vi "runnerFrontEnd.vi"(6 "ExperimentControlEvents":refnum<class "ExperimentControlEvents.lvclass">, 8 "error in (no error)":errorcluster, 9 "deviceDataBase":refnum<class "deviceDataBase.lvclass">, 10 "HWControllerEvents":refnum<class "HWControllerEvents.lvclass">, 11 "Views.lvlib:ExperimentControl.lvlib:ExperimentRunner in":refnum<class "ExperimentRunner.lvclass">) -> (0 "error out":errorcluster, 3 "Views.lvlib:ExperimentControl.lvlib:ExperimentRunner out":refnum<class "ExperimentRunner.lvclass">)   [LabVIEW 2009, in "Views.lvlib" / "ExperimentControl.lvlib" / "ExperimentRunner.lvclass"]
doc: "Experiment Runner Front End.\n\nThis is the user interface to control the expeirment. I.e. Run scripts and control the hardware state."
uses:
  ExperimentRunner.lvclass
  Hal/HWController/HWControllerEvents/HWControllerEvents.lvclass
  Tools/DatabaseHelpers/DbConnection/DeviceDataBase/deviceDataBase.lvclass
  Events/ExperimentControlEvents.lvclass
  ExperimentRunner.lvclass/ExperimentRunner.ctl
  Tools/SettingsProcessors/Compiler/Compiler.lvclass
  ScriptEditor/ScriptEditorV2/ScriptEditorV2.lvclass
  EventEditor/StaticOutputEditor/StaticOutputEditor.lvclass
  ScriptEditor/ScriptEdEvents/ScriptEdEvents.lvclass
  Tools/Filing/FileNeologist/FileNeologist.lvclass
  <vilib>/Utility/error.llb/DialogType.ctl
  Tools/DatabaseHelpers.lvlib
  Tools/Filing.lvlib
panel:
  in  "experimentFunction":enum16{"runListOnce", "loopOverList"}(ring)
  out "runningScriptName":string
  in  "HW Loop?":bool
  in  "refreshDatabase":bool
  in  "staticOutput":bool
  in  "stop":bool
  in  "runScript":bool
  in  "viewScript":bool
  in  "removePath":bool
  in  "addPath":bool
  out "status":T1(ring)
  in  "Listbox":i32(listbox)
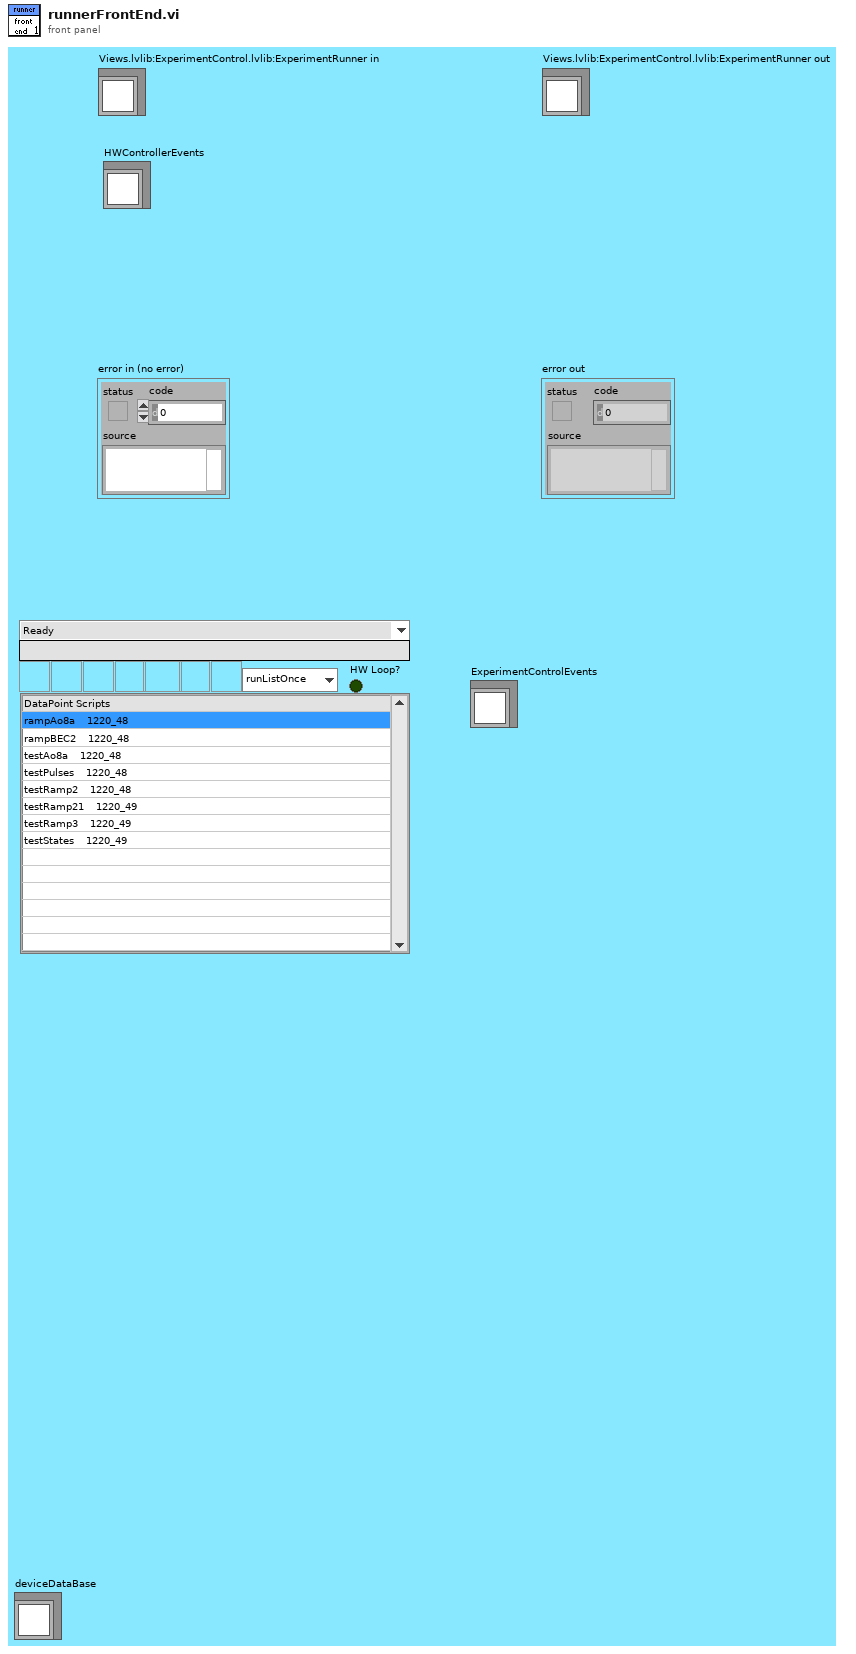
[diagram p1: front panel]
types:
  T1 = enum16{"Ready", "Compiling", "Configured", "Running", "Stopping", "Unresolved Error"}
  T2 = enum16{"start", "stop", "statusInquiry", "configure", "resetError", "resourcesInquiry", "reserveResources", "initialise", "resetAllChannels", "staticUpdate", "close", "HWStatus", "error", "resourcesAvailable", "resourcesReserved", "compilerError", "compiledScript", "compilingScript", "runScript", "configureCompiledScript"}
  T3 = enum16{"start", "stop", "statusInquiry", "configure", "resetError", "resourcesInquiry", "reserveResources", "initialise", "resetAllChannels", "staticUpdate", "close", "HWStatus", "error", "resourcesAvailable", "resourcesReserved"}
  T4 = enum16{"start", "stop", "statusInquiry", "configure", "resetError", "resourcesInquiry", "reserveResources", "initialise", "resetAllChannels", "staticUpdate", "close", "HWStatus", "error", "resourcesAvailable", "resourcesReserved", "compilerError", "compiledScript", "compilingScript", "runScript", "configureCompiledScript", "restartCompiler"}
  T5 = cluster{"incomingEventTypes":cluster{"start":cluster{"Boolean":bool}, "stop":cluster{"Boolean":bool}, "statusInquiry":cluster{"Boolean":bool}, "configure":cluster{"DPScriptPath":path, "TimeStamp":string, "HWLoop?":bool}, "resetError":cluster{"Boolean":bool}, "resourcesInquiry":cluster{"Boolean":bool}, "reserveResources":cluster{"HWList":string[]}, "initialise":cluster{"HWList":string[]}, "close":cluster{"Boolean":bool}, "resetAllChannels":cluster{"Boolean":bool}, "staticChannelUpdate":cluster{"channel_address":string, "calibratedValue":dbl}, "runScript":cluster{"DPScriptPath":path, "TimeStamp":string, "HWLoop?":bool}, "compilingScript":cluster{"Path":path}, "compiledScript":cluster{"Path":path, "timeCompileAt":string}, "compilerError":cluster{"Path":path}, "configureCompiledScript":cluster{"DPScriptPath":path, "TimeStamp":string, "HWLoop?":bool, "CompiledScript":cluster{"ScriptListCompiler.lvclass":refnum<class "ScriptListCompiler.lvclass">, "aoChannels":refnum<class "AnalogOutput.lvclass">[], "doChannels":refnum<class "DigitalOutput.lvclass">[], "rfChannels":refnum<class "DDSOutput.lvclass">[]}}, "restartCompiler":cluster{"restart":bool}, "staticRfChannelUpdate":cluster{"channel_address":string, "Output":cluster{"Frequency(MHz)":dbl, "Amplitude":dbl, "Phase":dbl, "OutputForm":enum16{"Sine", "Square", "Triangle", "Arbitrary"}}}}, "outgoingEventTypes":cluster{"HWStatus":cluster{"status":enum16{"Ready", "Compiling", "Configured", "Running", "Stopping", "Unresolved Error"}}, "error":cluster{"error out":errorcluster}, "resourcesAvailable":cluster{"availableHWList":string[], "reservedHWList":string[]}, "resourcesReserved":cluster{"reservedHWList":string[]}}}
  T6 = cluster{"open":cluster{"Path":path}, "close":cluster{"Boolean":bool}, "save":cluster{"Path":path}}
  T7 = cluster{"eventId":enum16{"Open", "Save", "Close"}, "close":cluster{"Boolean":bool}}
  T8 = cluster{"eventId":enum16{"start", "stop", "statusInquiry", "configure", "resetError", "resourcesInquiry", "reserveResources", "initialise", "resetAllChannels", "staticUpdate", "close", "HWStatus", "error", "resourcesAvailable", "resourcesReserved", "compilerError", "compiledScript", "compilingScript", "runScript", "configureCompiledScript"}, cluster{bool}}
  T9 = cluster{"eventId":enum16{"Open", "Save", "Close"}, "open":cluster{"Path":path}}
  T10 = typedef "eventsource.ctl" = u32
  T11 = enum16{"start", "stop", "statusInquiry", "configure", "resetError", "resourcesInquiry", "reserveResources", "initialise", "resetAllChannels", "staticUpdate", "close", "HWStatus", "error", "resourcesAvailable", "resourcesReserved", "compilerError", "compiledScript", "compilingScript", "runScript", "configureCompiledScript", "restartCompiler", "staticRfChannelUpdate"}
  T12 = cluster{"status":enum16{"Ready", "Compiling", "Configured", "Running", "Stopping", "Unresolved Error"}}
  T13 = typedef "DialogType.ctl" = u16
  T14 = cluster{"eventId":enum16{"start", "stop", "statusInquiry", "configure", "resetError", "resourcesInquiry", "reserveResources", "initialise", "resetAllChannels", "staticUpdate", "close", "HWStatus", "error", "resourcesAvailable", "resourcesReserved"}, "resetError":cluster{"Boolean":bool}}
  T15 = cluster{"eventId":enum16{"start", "stop", "statusInquiry", "configure", "resetError", "resourcesInquiry", "reserveResources", "initialise", "resetAllChannels", "staticUpdate", "close", "HWStatus", "error", "resourcesAvailable", "resourcesReserved"}, cluster{bool}}
  T16 = typedef "LVPoint32TypeDef.ctl" = cluster{"Horizontal":i32, "Vertical":i32}
  T17 = cluster{"eventId":enum16{"start", "stop", "statusInquiry", "configure", "resetError", "resourcesInquiry", "reserveResources", "initialise", "resetAllChannels", "staticUpdate", "close", "HWStatus", "error", "resourcesAvailable", "resourcesReserved", "compilerError", "compiledScript", "compilingScript", "runScript", "configureCompiledScript", "restartCompiler"}, cluster{bool}}
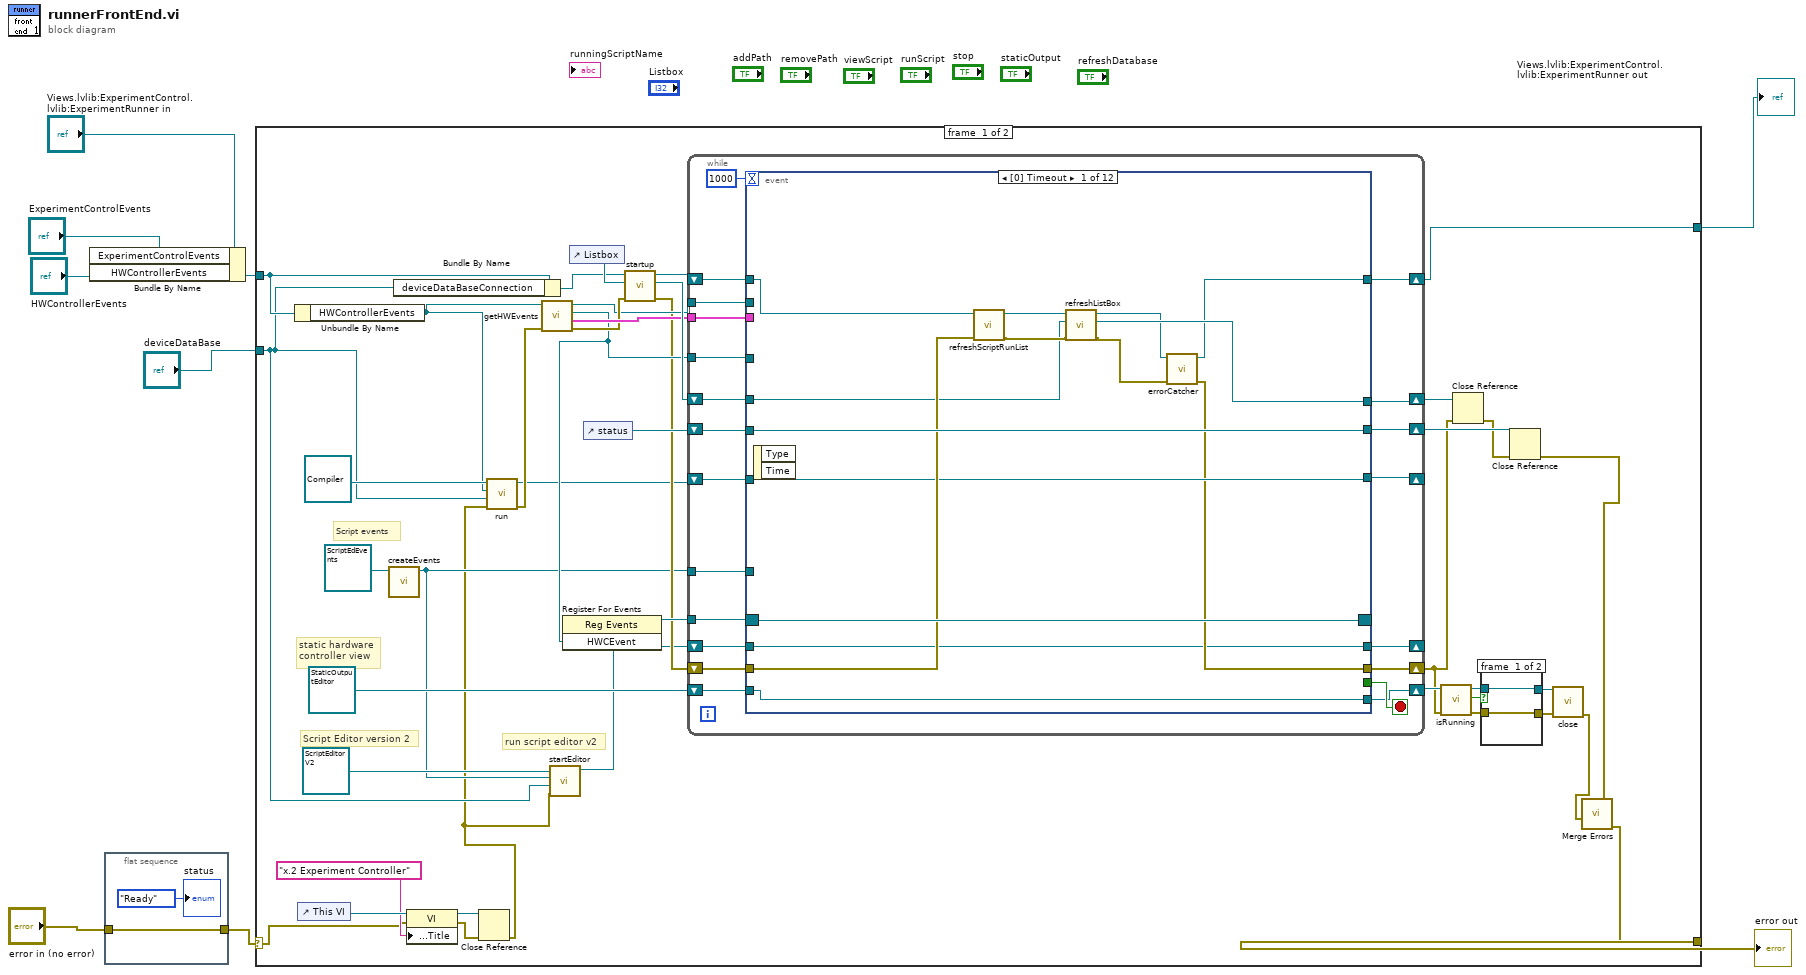
[diagram p0: block diagram]
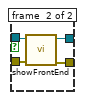
[diagram p2: hidden frame]
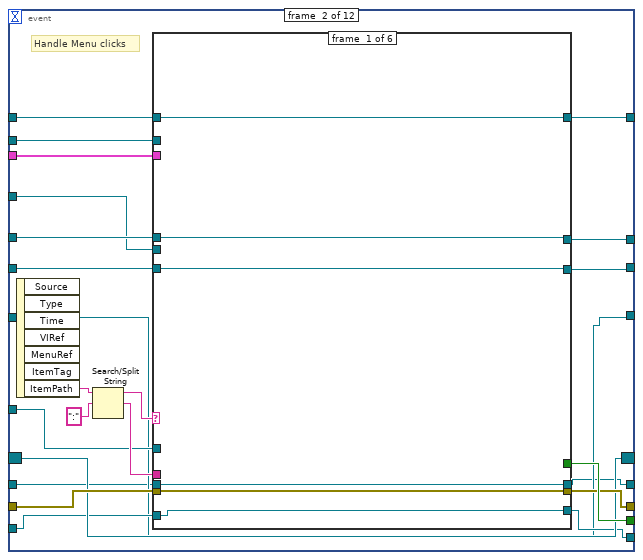
[diagram p3: hidden frame]
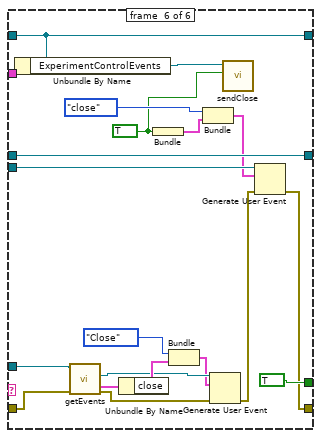
[diagram p9: hidden frame]
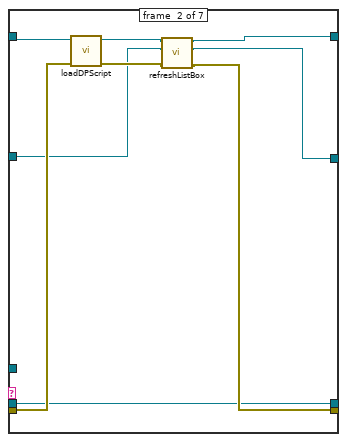
[diagram p17: hidden frame]
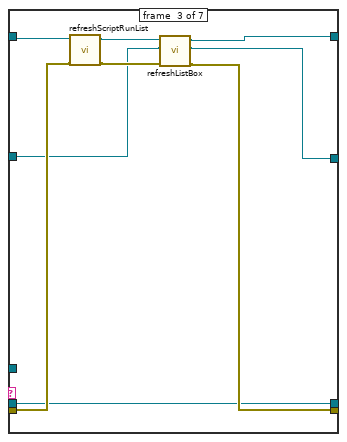
[diagram p18: hidden frame]
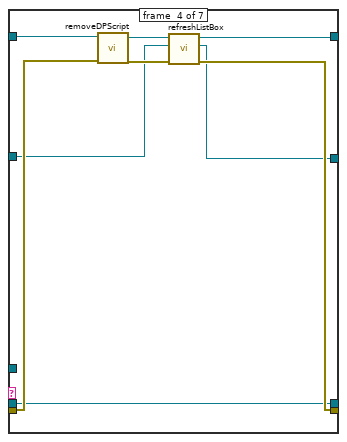
[diagram p19: hidden frame]
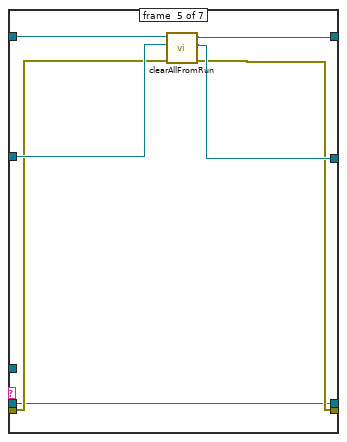
[diagram p20: hidden frame]
diagram:
  n1 = Bundle By Name(cluster="Views.lvlib:ExperimentControl.lvlib:ExperimentRunner in", "ExperimentControlEvents"="ExperimentControlEvents", "HWControllerEvents"="HWControllerEvents") -> (w5:refnum<class "ExperimentRunner.lvclass">)
  n2 = flat-sequence {
    tunnel: "error in (no error)" -> [w10]
    tunnel: [w10] -> w2
    frame #0 {
      "status" <- T1."Ready" ("status")
    }
  }
  n3 = case shown="No Error" w2 {
    selector: w2 -> [w28 w688]
    tunnel: [w41 w688] -> w9
    tunnel: [w32 w687] -> w8
    tunnel: w5 -> [w36 w687]
    tunnel: "deviceDataBase" -> [w14 _]
    frame #0 {
      # "run script editor v2"
      # "Script Editor version 2"
      # "Script events"
      # "static hardware\ncontroller view"
      n4 = Unbundle By Name(w36) -> ("HWControllerEvents"=w29:refnum<class "HWControllerEvents.lvclass">)
      n5 = control-ref of="This VI"() -> (w40:refnum<vi>)
      n6 = call-dynamic "createEvents.vi"("ScriptEdEvents in"=refnum<class "ScriptEdEvents.lvclass"> refnum ("Views.lvlib:SciptEditor.lvlib:ScriptEdEvents.lvclass")) -> ("ScriptEdEvents out"=w15:refnum<class "ScriptEdEvents.lvclass">)  [unwired: 9 in, 1 out]
      n7 = Bundle By Name(cluster=w36, "deviceDataBaseConnection"=w14) -> (w35:refnum<class "ExperimentRunner.lvclass">)
      n8 = property class="VI"(reference=w40, error in=w28, "Front Panel.Title"="x.2 Experiment Controller") -> (reference out=w38:refnum<vi>, error out=w37:errorcluster)
      n9 = Close Reference(reference=w38, error in (no error)=w37) -> (error out=w13:errorcluster)
      n10 = call "run.vi"("error in (no error)"=w13, "deviceDataBase"=w14, "HWControllerEvents"=w29, "Compiler in"=refnum<class "Compiler.lvclass"> refnum) -> ("error out"=w27:errorcluster, "Compiler out"=w26:refnum<class "Compiler.lvclass">)  [unwired: 6 in]
      n11 = call-dynamic "getHWEvents.vi"("error in (no error)"=w27, "HWControllerEvents in"=w29) -> ("error out"=w47:errorcluster, "eventDataTypes"=w48:T5, "HWCEvent"=w46:refnum<user-event>, "HWControllerEvents out"=w34:refnum<class "HWControllerEvents.lvclass">)  [unwired: 6 in]
      n12 = call "startEditor.vi"("error in (no error)"=w13, "deviceDataBase"=w14, "ScriptEdEvents"=w15, "ScriptEditorV2 in"=refnum<class "ScriptEditorV2.lvclass"> refnum ("Views.lvlib:SciptEditor.lvlib:ScriptEditorV2.lvclass")) -> ("ScriptEditorV2 out"=w12:refnum<class "ScriptEditorV2.lvclass">)  [unwired: 6 in, 1 out]
      n13 = register-events(w46) -> (reference out=w49:refnum<event-registration>)  [unwired: 2 in, 1 out]
      n14 = control-ref of="Listbox"() -> (w51:refnum<vi>)
      n15 = control-ref of="status"() -> (w45:refnum<vi>)
      n16 = call "startup.vi"("error in (no error)"=w47, "Listbox in"=w51, "ExperimentRunner in"=w35) -> ("error out"=w31:errorcluster, "Listbox out"=w50:refnum<vi>, "ExperimentRunner out"=w52:refnum<class "ExperimentRunner.lvclass">)  [unwired: 6 in]
      n17 = while {
        shift-right: [w79] -> w32
        shift-left: w52 -> [w66]
        shift-right: [w78] -> w24
        shift-left: w31 -> [w65]
        shift-right: [w77] -> w53
        shift-left: w50 -> [w67]
        tunnel: w49 -> [w76]
        tunnel: w48 -> [w75]
        tunnel: w46 -> [w74]
        shift-right: [w72] -> w44
        shift-left: w45 -> [w73]
        tunnel: w15 -> [w71]
        tunnel: w34 -> [w70]
        shift-right: [w68] -> w25
        shift-left: refnum<class "StaticOutputEditor.lvclass"> refnum ("Views.lvlib:SciptEditor.lvlib:StaticOutputEditor.lvclass") -> [w69]
        shift-right: [w62] -> _
        shift-left: w26 -> [w63]
        shift-right: [w61] -> _
        shift-left: w12 -> [w60]
        stop <- w80 stop-if-true
        n18 = event shown="[0] Timeout" {
          selector: w76 -> [w94 w107 w389 _ _ w564 w577 w584 w618 w631 w639 w675]
          dyn-events: [w94 w107 w389 _ _ w564 w577 w584 w618 w631 w639 w675] -> _
          timeout: 1000 -> [_ _ _ _ _ _ _ _ _ _ _ _]
          tunnel: [_ w118 _ TRUE _ _ _ _ _ _ _ _] -> w80
          tunnel: w66 -> [w92 w113 w383 w518 w547 w568 w581 w596 w614 w625 w646 w685]
          tunnel: [w82 w112 w382 w517 w546 w562 w575 w596 w613 w624 w646 w684] -> w79
          tunnel: [w84 w110 w390 w522 w554 w558 w571 w592 w611 w626 w644 w664] -> w78
          tunnel: w65 -> [w91 w111 w391 w521 w543 w565 w579 w594 w615 w627 w635 w673]
          tunnel: w67 -> [w88 w109 w381 w538 w548 w561 w574 w595 w620 w630 w641 w682]
          tunnel: [w87 w108 w380 w538 w548 w560 w573 w595 w620 w630 w641 w682] -> w77
          tunnel: w75 -> [_ w106 w392 _ _ _ _ _ _ _ _ _]
          tunnel: w74 -> [_ w105 w385 w524 _ _ _ _ _ _ _ w679]
          tunnel: w73 -> [w95 w104 w388 w537 w544 w567 w580 w585 w612 w629 w640 w681]
          tunnel: [w95 w103 w387 w537 w544 w567 w580 w585 w612 w629 w640 w681] -> w72
          tunnel: w71 -> [_ w102 _ w523 _ _ _ w593 _ _ _ _]
          tunnel: w70 -> [_ w101 _ _ _ _ _ _ _ _ w645 _]
          tunnel: w69 -> [w93 w100 w384 w536 w542 w566 w578 w591 w619 w628 w637 w683]
          tunnel: [w93 w99 w384 w536 w542 w566 w578 w591 w619 w628 w643 w683] -> w68
          tunnel: w63 -> [w86 w98 w379 w515 w541 w557 w570 w583 w610 w622 w638 w668]
          tunnel: [w86 w98 w379 w515 w541 w557 w570 w583 w610 w622 w638 w665] -> w62
          tunnel: [w81 w96 w378 w514 w540 w556 w569 w582 w609 w621 w632 w663] -> w61
          tunnel: w60 -> [w81 w97 w378 w514 w540 w556 w569 w582 w609 w621 w632 w663]
          event #0 {
            n19 = event-data() -> ()  [unwired: 1 in, 2 out]
            n20 = call "refreshScriptRunList.vi"("error in (no error)"=w91, "ExperimentRunner in"=w92) -> ("error out"=w90:errorcluster, "ExperimentRunner out"=w89:refnum<class "ExperimentRunner.lvclass">)  [unwired: 8 in]
            n21 = call "refreshListBox.vi"("error in (no error)"=w90, "Listbox"=w88, "ExperimentRunner in"=w89) -> ("error out"=w85:errorcluster, "Listbox out"=w87:refnum<vi>, "ExperimentRunner out"=w83:refnum<class "ExperimentRunner.lvclass">)  [unwired: 6 in]
            n22 = call "errorCatcher.vi"("error in (no error)"=w85, "ExperimentRunner in"=w83) -> ("error out"=w84:errorcluster, "ExperimentRunner out"=w82:refnum<class "ExperimentRunner.lvclass">)  [unwired: 8 in]
          }
          event #1 {
            # "Handle Menu clicks"
            n23 = event-data() -> ("ItemPath"=w116:string)  [unwired: 1 in, 6 out]
            n24 = Search/Split String(string=w116, search string/char (-)=":") -> (substring before match=w115:string, match + rest of string=w114:string)  [unwired: 1 in, 1 out]
            n25 = case shown="\"Scripting\"" w115 {
              tunnel: [_ w138 _ _ _ _] -> w118
              tunnel: w114 -> [_ w137 w178 w208 w299 w349]
              tunnel: w113 -> [w124 w136 w182 w212 w303 w348]
              tunnel: [w124 w135 w181 w211 w302 w347] -> w112
              tunnel: w111 -> [w123 w134 w179 w209 w300 w346]
              tunnel: [w123 w133 w180 w210 w301 w345] -> w110
              tunnel: w109 -> [w122 w132 w177 w207 w298 w344]
              tunnel: [w122 w131 w176 w206 w297 w344] -> w108
              tunnel: w106 -> [_ w130 _ _ _ _]
              tunnel: w105 -> [_ w129 _ _ _ w342]
              tunnel: w104 -> [w121 w128 w175 w205 w296 w343]
              tunnel: [w121 w128 w175 w205 w295 w343] -> w103
              tunnel: w102 -> [_ w127 _ w204 _ _]
              tunnel: w101 -> [_ _ _ _ _ w341]
              tunnel: w100 -> [w120 w126 w174 w203 w294 w340]
              tunnel: [w120 w126 w174 w203 w294 w339] -> w99
              tunnel: w97 -> [w119 w125 w173 w202 w293 w338]
              tunnel: [w119 w125 w173 w201 w293 w338] -> w96
              frame #0 {
              }
              frame #1 {
                n26 = case shown="\":Close\"" w137 {
                  tunnel: [_ _ _ _ _ TRUE] -> w138
                  tunnel: [w141 w144 w147 w150 w153 w156] -> w135
                  tunnel: w136 -> [w141 w144 w147 w150 w153 w156]
                  tunnel: w134 -> [w140 w143 w146 w149 w152 w158]
                  tunnel: [w140 w143 w146 w149 w152 w167] -> w133
                  tunnel: w132 -> [w139 w142 w145 w148 w151 w171]
                  tunnel: [w139 w142 w145 w148 w151 w171] -> w131
                  tunnel: w130 -> [_ _ _ _ _ _]
                  tunnel: w129 -> [_ _ _ _ _ w170]
                  tunnel: w127 -> [_ _ _ _ _ w166]
                  frame #0 {
                  }
                  frame #1 {
                  }
                  frame #2 {
                  }
                  frame #3 {
                  }
                  frame #4 {
                  }
                  frame #5 {
                    w154 = TRUE
                    n27 = Unbundle By Name(w156) -> ("ExperimentControlEvents"=w155:refnum<class "ExperimentControlEvents.lvclass">)
                    n28 = call-dynamic "getEvents.vi"("error in (no error)"=w158, "ScriptEdEvents in"=w166) -> ("error out"=w160:errorcluster, "eventsToScriptEd"=w165:T6, "ScriptEvent"=w162:refnum<user-event>)  [unwired: 6 in, 1 out]
                    n29 = Unbundle By Name(w165) -> ("close"=w163:cluster{"Boolean":bool})
                    n30 = Bundle(w154) -> (w169:cluster{bool})  [unwired: 1 in]
                    n31 = Bundle("eventId"=enum16{"Open", "Save", "Close"}."Close", "close"=w163) -> (w161:T7)  [unwired: 1 in]
                    n32 = Bundle("eventId"=T2."close", w169) -> (w168:T8)  [unwired: 1 in]
                    n33 = Generate User Event(user event=w162, event data cluster=w161, error in=w160) -> (error out=w159:errorcluster)  [unwired: 1 out]
                    n34 = call "sendClose.vi"("close"=w154, "ExperimentControlEvents in"=w155) -> ()  [unwired: 8 in, 2 out]
                    n35 = Generate User Event(user event=w170, event data cluster=w168, error in=w159) -> (error out=w167:errorcluster)  [unwired: 1 out]
                  }
                }
              }
              frame #2 {
                n36 = case shown="\":Paste\"" w178 {
                  tunnel: [w185 w188 w191 w194 w197 w200] -> w181
                  tunnel: w182 -> [w185 w188 w191 w194 w197 w200]
                  tunnel: [w184 w187 w190 w193 w196 w199] -> w180
                  tunnel: w179 -> [w184 w187 w190 w193 w196 w199]
                  tunnel: w177 -> [w183 w186 w189 w192 w195 w198]
                  tunnel: [w183 w186 w189 w192 w195 w198] -> w176
                  frame #0 {
                  }
                  frame #1 {
                  }
                  frame #2 {
                  }
                  frame #3 {
                  }
                  frame #4 {
                  }
                  frame #5 {
                  }
                }
              }
              frame #3 {
                n37 = case shown="\":Open Script Editor\"" w208 {
                  tunnel: [w216 w221 w229 w239 w246 w260 w276] -> w211
                  tunnel: w212 -> [w216 w225 w234 w243 w250 w260 w276]
                  tunnel: [w215 w218 w231 w240 w245 w255 w278] -> w210
                  tunnel: w209 -> [w215 w224 w233 w242 w248 w256 w282]
                  tunnel: w207 -> [w214 w220 w228 w237 w249 w261 w284]
                  tunnel: [w214 w219 w227 w236 w247 w261 w284] -> w206
                  tunnel: w204 -> [_ _ _ _ _ w257 w274]
                  tunnel: w202 -> [w213 w217 w226 w235 w244 w251 w283]
                  tunnel: [w213 w217 w226 w235 w244 w251 w280] -> w201
                  frame #0 {
                  }
                  frame #1 {
                    n38 = call "loadDPScript.vi"("error in (no error)"=w224, "ExperimentRunner in"=w225) -> ("error out"=w223:errorcluster, "ExperimentRunner out"=w222:refnum<class "ExperimentRunner.lvclass">)  [unwired: 8 in]
                    n39 = call "refreshListBox.vi"("error in (no error)"=w223, "Listbox"=w220, "ExperimentRunner in"=w222) -> ("error out"=w218:errorcluster, "Listbox out"=w219:refnum<vi>, "ExperimentRunner out"=w221:refnum<class "ExperimentRunner.lvclass">)  [unwired: 6 in]
                  }
                  frame #2 {
                    n40 = call "refreshScriptRunList.vi"("error in (no error)"=w233, "ExperimentRunner in"=w234) -> ("error out"=w232:errorcluster, "ExperimentRunner out"=w230:refnum<class "ExperimentRunner.lvclass">)  [unwired: 8 in]
                    n41 = call "refreshListBox.vi"("error in (no error)"=w232, "Listbox"=w228, "ExperimentRunner in"=w230) -> ("error out"=w231:errorcluster, "Listbox out"=w227:refnum<vi>, "ExperimentRunner out"=w229:refnum<class "ExperimentRunner.lvclass">)  [unwired: 6 in]
                  }
                  frame #3 {
                    n42 = call "removeDPScript.vi"("error in (no error)"=w242, "ExperimentRunner in"=w243) -> ("error out"=w241:errorcluster, "ExperimentRunner out"=w238:refnum<class "ExperimentRunner.lvclass">)  [unwired: 8 in]
                    n43 = call "refreshListBox.vi"("error in (no error)"=w241, "Listbox"=w237, "ExperimentRunner in"=w238) -> ("error out"=w240:errorcluster, "Listbox out"=w236:refnum<vi>, "ExperimentRunner out"=w239:refnum<class "ExperimentRunner.lvclass">)  [unwired: 6 in]
                  }
                  frame #4 {
                    n44 = call "clearAllFromRun.vi"("error in (no error)"=w248, "Listbox in"=w249, "ExperimentRunner in"=w250) -> ("error out"=w245:errorcluster, "Listbox out"=w247:refnum<vi>, "ExperimentRunner out"=w246:refnum<class "ExperimentRunner.lvclass">)  [unwired: 6 in]
                  }
                  frame #5 {
                    # "send open event to script editor"
                    n45 = Unbundle By Name(w260) -> ("scriptSelected"=w258:i32, "PathArray"=w259:path[])
                    n46 = Index Array(array=w259, index=w258) -> (element=w254:path)
                    n47 = Equal?(x=w254, y=path "") -> (x = y?=w252:bool)
                    n48 = case shown="False" w252 {
                      tunnel: w257 -> [w272 _]
                      tunnel: w256 -> [w271 w273]
                      tunnel: [w263 w273] -> w255
                      tunnel: w254 -> [w262 _]
                      frame #0 {
                        n49 = call-dynamic "getEvents.vi"("error in (no error)"=w271, "ScriptEdEvents in"=w272) -> ("error out"=w264:errorcluster, "eventsToScriptEd"=w270:T6, "ScriptEvent"=w268:refnum<user-event>)  [unwired: 6 in, 1 out]
                        n50 = Unbundle By Name(w270) -> ("open"=w269:cluster{"Path":path})
                        n51 = Bundle By Name(cluster=w269, "Path"=w262) -> (w266:cluster{"Path":path})
                        n52 = Bundle("eventId"=enum16{"Open", "Save", "Close"}."Open", "open"=w266) -> (w265:T9)  [unwired: 1 in]
                        n53 = Generate User Event(user event=w268, event data cluster=w265, error in=w264) -> (error out=w263:errorcluster)  [unwired: 1 out]
                      }
                      frame #1 {
                      }
                    }
                  }
                  frame #6 {
                    n54 = Unbundle By Name(w276) -> ("deviceDataBaseConnection"=w275:refnum<class "deviceDataBase.lvclass">)
                    n55 = call "isRunning.vi"("error in (no error)"=w282, "ScriptEditorV2 in"=w283) -> ("error out"=w277:errorcluster, "Running?"=w281:bool, "ScriptEditorV2 out"=w279:refnum<class "ScriptEditorV2.lvclass">)  [unwired: 7 in]
                    n56 = case shown="False" w281 {
                      tunnel: [w288 w292] -> w280
                      tunnel: w279 -> [w290 w292]
                      tunnel: [w287 w291] -> w278
                      tunnel: w277 -> [w289 w291]
                      tunnel: w275 -> [w286 _]
                      tunnel: w274 -> [w285 _]
                      frame #0 {
                        n57 = call "startEditor.vi"("error in (no error)"=w289, "deviceDataBase"=w286, "ScriptEdEvents"=w285, "ScriptEditorV2 in"=w290) -> ("error out"=w287:errorcluster, "ScriptEditorV2 out"=w288:refnum<class "ScriptEditorV2.lvclass">)  [unwired: 6 in]
                      }
                      frame #1 {
                      }
                    }
                  }
                }
              }
              frame #4 {
                n58 = case shown="\":Pause Experiment\"" w299 {
                  tunnel: [w307 w313 w320 w327 w334] -> w302
                  tunnel: w303 -> [w307 w314 w322 w328 w335]
                  tunnel: [w306 w308 w318 w325 w333] -> w301
                  tunnel: w300 -> [w306 w310 w319 w326 w332]
                  tunnel: w298 -> [w305 w315 w323 w330 w337]
                  tunnel: [w305 w315 w323 w330 w337] -> w297
                  tunnel: w296 -> [w304 w309 w317 w329 w336]
                  tunnel: [w304 w309 w317 w329 w336] -> w295
                  frame #0 {
                  }
                  frame #1 {
                    n59 = Unbundle By Name(w314) -> ("scriptSelected"=w312:i32)
                    n60 = local read "HW Loop?"() -> (w311:bool)
                    n61 = call "runSingleScriptV3.vi"("error in (no error)"=w310, "HWLoop"=w311, "index"=w312, "ExperimentRunner in"=w314) -> ("error out"=w308:errorcluster, "ExperimentRunner out"=w313:refnum<class "ExperimentRunner.lvclass">)  [unwired: 6 in]
                  }
                  frame #2 {
                    n62 = Unbundle By Name(w322) -> ("scriptSelected"=w321:i32)
                    n63 = call "runExperimentV2.vi"("error in (no error)"=w319, "runExperiment.Enum"="experimentFunction", "index"=w321, "ExperimentRunner in"=w322) -> ("error out"=w318:errorcluster, "ExperimentRunner out"=w320:refnum<class "ExperimentRunner.lvclass">)  [unwired: 6 in]
                  }
                  frame #3 {
                    n64 = call "sendStop.vi"("error in (no error)"=w326, "stop"=enum16{"stopBeforeNext", "stopNow"}."stopBeforeNext", "ExperimentRunner in"=w328) -> ("error out"=w325:errorcluster, "ExperimentRunner out"=w327:refnum<class "ExperimentRunner.lvclass">)  [unwired: 7 in]
                  }
                  frame #4 {
                    n65 = call "sendStop.vi"("error in (no error)"=w332, "stop"=enum16{"stopBeforeNext", "stopNow"}."stopNow", "ExperimentRunner in"=w335) -> ("error out"=w333:errorcluster, "ExperimentRunner out"=w334:refnum<class "ExperimentRunner.lvclass">)  [unwired: 7 in]
                  }
                }
              }
              frame #5 {
                n66 = case shown="\":Update Channel Output\"" w349 {
                  tunnel: w348 -> [w352 w362]
                  tunnel: [w352 w362] -> w347
                  tunnel: w346 -> [w351 w355]
                  tunnel: [w351 w359] -> w345
                  tunnel: w342 -> [_ _]
                  tunnel: w341 -> [_ w361]
                  tunnel: w340 -> [w350 w354]
                  tunnel: [w350 w360] -> w339
                  frame #0 {
                  }
                  frame #1 {
                    n67 = Unbundle By Name(w362) -> ("deviceDataBaseConnection"=w358:refnum<class "deviceDataBase.lvclass">)
                    n68 = call "isRunning.vi"("error in (no error)"=w355, "StaticOutputEditor in"=w354) -> ("error out"=w356:errorcluster, "running?"=w353:bool, "StaticOutputEditor out"=w357:refnum<class "StaticOutputEditor.lvclass">)  [unwired: 7 in]
                    n69 = case shown="False" w353 {
                      tunnel: w357 -> [w373 w377]
                      tunnel: w361 -> [w371 _]
                      tunnel: [w370 w375] -> w360
                      tunnel: [w369 w374] -> w359
                      tunnel: w358 -> [w368 _]
                      tunnel: w356 -> [w366 w376]
                      frame #0 {
                        n70 = call "close.vi"("error in (no error)"=w366, "StaticOutputEditor in"=w373) -> ("error out"=w365:errorcluster, "StaticOutputEditor out"=w372:refnum<class "StaticOutputEditor.lvclass">)  [unwired: 8 in]
                        n71 = call "getUnrestrictedChannelArray.vi"("error in (no error)"=w366, "deviceDataBase in"=w368) -> ("error out"=w364:errorcluster, "ChannelArray.lvclass"=w367:refnum<class "ChannelArray.lvclass">)  [unwired: 7 in, 1 out]
                        n72 = call <vilib>:"Merge Errors.vi"("error in 2 (no error)"=w364, "error in 1 (no error)"=w365) -> ("error out"=w363:errorcluster)  [unwired: 5 in]
                        n73 = call-dynamic "run.vi"("error in (no error)"=w363, "HWControllerEvents"=w371, "ChannelArray"=w367, "StaticOutputEditor"=w372) -> ("error out"=w369:errorcluster, "StaticOutputEditor out"=w370:refnum<class "StaticOutputEditor.lvclass">)  [unwired: 6 in]
                      }
                      frame #1 {
                        n74 = call "showFrontEnd.vi"("error in (no error)"=w376, "StaticOutputEditor in"=w377) -> ("error out"=w374:errorcluster, "StaticOutputEditor out"=w375:refnum<class "StaticOutputEditor.lvclass">)  [unwired: 8 in]
                      }
                    }
                  }
                }
              }
            }
          }
          event #2 {
            # "recieve hardware events."
            n75 = event-data() -> ("Source"=w386:T10, "eventId"=w394:T11, "data"=w393:variant)  [unwired: 1 in, 3 out]
            n76 = case shown="\"HWStatus\"" w394 {
              tunnel: w393 -> [_ w410 w421 w451 w466 w501 _ _]
              tunnel: w392 -> [_ w409 w428 w460 w474 w499 _ _]
              tunnel: w391 -> [w397 w407 w420 w446 w462 w500 w509 w513]
              tunnel: [w397 w402 w425 w457 w471 w487 w509 w513] -> w390
              tunnel: w388 -> [w398 w404 w422 w454 w468 w496 w508 w512]
              tunnel: [w398 w403 w422 w454 w468 w494 w508 w512] -> w387
              tunnel: w386 -> [_ _ _ _ _ _ _ _]
              tunnel: w385 -> [_ _ _ _ _ w493 _ _]
              tunnel: w383 -> [w396 w401 w427 w459 w473 w477 w507 w511]
              tunnel: [w396 w401 w426 w458 w472 w477 w507 w511] -> w382
              tunnel: w381 -> [w395 w400 w424 w456 w470 w476 w506 w510]
              tunnel: [w395 w400 w423 w455 w469 w476 w506 w510] -> w380
              frame #0 {
              }
              frame #1 {
                n77 = Unbundle By Name(w409) -> ("outgoingEventTypes.HWStatus"=w408:T12)
                n78 = Variant To Data(error in=w407, Variant=w410, type=w408) -> (error out=w406:errorcluster, data=w405:T12)
                n79 = Unbundle By Name(w405) -> ("status"=w399:T1)
                n80 = case shown="\"Running\"" w399 {
                  frame #0 {
                    n81 = local write "runningScriptName"("") -> ()
                  }
                  frame #1 {
                    n82 = local write "runningScriptName"("") -> ()
                  }
                  frame #2 {
                    n83 = call "globalFileNeologist.vi"("Action"=enum16{"Write", "Read"}."Read") -> ("FileNeologist out"=w418:refnum<class "FileNeologist.lvclass">)  [unwired: 10 in]
                    n84 = call <vilib>:"Space Constant.vi"() -> ("String"=w414:string)
                    n85 = call-dynamic "getScriptName.vi"("FileNeologist.lvclass in"=w418) -> ("scriptName"=w415:string, "FileNeologist.lvclass out"=w417:refnum<class "FileNeologist.lvclass">)  [unwired: 8 in, 1 out]
                    n86 = call "getTimeStamp.vi"("FileNeologist in"=w417) -> ("TimeStamp"=w416:string)  [unwired: 8 in, 2 out]
                    n87 = Concatenate Strings(w416, w414, w415) -> (w413:string)
                    n88 = local write "runningScriptName"(w413) -> ()
                  }
                  frame #3 {
                  }
                  frame #4 {
                  }
                }
                n89 = property class="Enum (strict)"(reference=w404, error in=w406, "Value"=w399) -> (reference out=w403:refnum<vi>, error out=w402:errorcluster)
              }
              frame #2 {
                n90 = disable-structure shown="Enabled" {
                  disable-tunnel: w428 -> [w441 _]
                  disable-tunnel: w427 -> [w440 w444]
                  disable-tunnel: [w439 w444] -> w426
                  disable-tunnel: [w438 w442] -> w425
                  disable-tunnel: w424 -> [w437 w443]
                  disable-tunnel: [w436 w443] -> w423
                  disable-tunnel: w421 -> [w434 _]
                  disable-tunnel: w420 -> [w430 w442]
                  frame #0 {
                    n91 = Unbundle By Name(w441) -> ("incomingEventTypes.compilerError"=w433:cluster{"Path":path})
                    n92 = Variant To Data(error in=w430, Variant=w434, type=w433) -> (error out=w429:errorcluster, data=w432:cluster{"Path":path})
                    n93 = Unbundle By Name(w432) -> ("Path"=w431:path)
                    n94 = call "compilerUpdate.vi"("String"="    Compiler Error", "error in (no error)"=w429, "Path"=w431, "Listbox in"=w437, "ExperimentRunner in"=w440) -> ("error out"=w438:errorcluster, "Listbox out"=w436:refnum<vi>, "ExperimentRunner out"=w439:refnum<class "ExperimentRunner.lvclass">)  [unwired: 4 in]
                  }
                  frame #1 {
                  }
                }
              }
              frame #3 {
                n95 = Unbundle By Name(w460) -> ("incomingEventTypes.compiledScript"=w450:cluster{"Path":path, "timeCompileAt":string})
                n96 = Variant To Data(error in=w446, Variant=w451, type=w450) -> (error out=w445:errorcluster, data=w449:cluster{"Path":path, "timeCompileAt":string})
                n97 = Unbundle By Name(w449) -> ("timeCompileAt"=w448:string, "Path"=w447:path)
                n98 = Concatenate Strings("    ", w448) -> (w452:string)
                n99 = call "compilerUpdate.vi"("String"=w452, "error in (no error)"=w445, "Path"=w447, "Listbox in"=w456, "ExperimentRunner in"=w459) -> ("error out"=w457:errorcluster, "Listbox out"=w455:refnum<vi>, "ExperimentRunner out"=w458:refnum<class "ExperimentRunner.lvclass">)  [unwired: 4 in]
              }
              frame #4 {
                n100 = Unbundle By Name(w474) -> ("incomingEventTypes.compilingScript"=w465:cluster{"Path":path})
                n101 = Variant To Data(error in=w462, Variant=w466, type=w465) -> (error out=w461:errorcluster, data=w463:cluster{"Path":path})
                n102 = Unbundle By Name(w463) -> ("Path"=w464:path)
                n103 = call "compilerUpdate.vi"("String"="    Compiling", "error in (no error)"=w461, "Path"=w464, "Listbox in"=w470, "ExperimentRunner in"=w473) -> ("error out"=w471:errorcluster, "Listbox out"=w469:refnum<vi>, "ExperimentRunner out"=w472:refnum<class "ExperimentRunner.lvclass">)  [unwired: 4 in]
              }
              frame #5 {
                w475 = T13 1 items=["no dialog", "OK message", "continue or stop message", "OK message + warnings", "continue/stop + warnings"] ("type of dialog (OK msg:1)")
                w482 = "\r\n"
                n104 = Unbundle By Name(w499) -> ("incomingEventTypes.resetError"=w492:cluster{"Boolean":bool}, "outgoingEventTypes.error"=w498:cluster{"error out":errorcluster})
                n105 = Variant To Data(error in=w500, Variant=w501, type=w498) -> (error out=w495:errorcluster, data=w497:cluster{"error out":errorcluster})
                n106 = Unbundle By Name(w497) -> ("error out"=w484:errorcluster)
                n107 = Bundle By Name(cluster=w492, "Boolean"=TRUE) -> (w490:cluster{"Boolean":bool})
                n108 = Unbundle By Name(w484) -> ("source"=w481:string)
                n109 = property class="Enum (strict)"(reference=w496, error in=w495, "Value"=T1."Unresolved Error") -> (reference out=w494:refnum<vi>, error out=w488:errorcluster)
                n110 = Bundle("eventId"=T3."resetError", "resetError"=w490) -> (w489:T14)  [unwired: 1 in]
                n111 = Concatenate Strings(w481, w482, w482, "\nA hardware error has occured with the above code. Clicking ok will clear the error, however restarting the program or labview may be necessary depending on the problem.") -> (w485:string)
                n112 = Bundle By Name(cluster=w484, "source"=w485) -> (w483:errorcluster)
                n113 = flat-sequence {
                  tunnel: w493 -> [w505]
                  tunnel: w489 -> [w504]
                  tunnel: w488 -> [w503]
                  tunnel: [w502] -> w487
                  tunnel: w486 -> [_]
                  frame #0 {
                    n114 = Generate User Event(user event=w505, event data cluster=w504, error in=w503) -> (error out=w502:errorcluster)  [unwired: 1 out]
                  }
                }
                n115 = call <vilib>:"Simple Error Handler.vi"("type of dialog (OK msg:1)"=w475, "error in (no error)"=w483) -> ("error out"=w486:errorcluster)  [unwired: 3 in, 4 out]
              }
              frame #6 {
              }
              frame #7 {
              }
            }
          }
          event #3 {
            # "close"
            n116 = event-data() -> ()  [unwired: 1 in, 4 out]
            n117 = Unbundle By Name(w518) -> ("ExperimentControlEvents"=w520:refnum<class "ExperimentControlEvents.lvclass">)
            n118 = call-dynamic "getEvents.vi"("error in (no error)"=w521, "ScriptEdEvents in"=w523) -> ("error out"=w527:errorcluster, "eventsToScriptEd"=w532:T6, "ScriptEvent"=w529:refnum<user-event>)  [unwired: 6 in, 1 out]
            n119 = Unbundle By Name(w532) -> ("close"=w530:cluster{"Boolean":bool})
            n120 = Bundle(TRUE) -> (w534:cluster{bool})  [unwired: 1 in]
            n121 = call "sendClose.vi"("close"=TRUE, "ExperimentControlEvents in"=w520) -> ("ExperimentControlEvents out"=w516:refnum<class "ExperimentControlEvents.lvclass">)  [unwired: 8 in, 1 out]
            n122 = Bundle("eventId"=enum16{"Open", "Save", "Close"}."Close", "close"=w530) -> (w528:T7)  [unwired: 1 in]
            n123 = Bundle("eventId"=T3."close", w534) -> (w533:T15)  [unwired: 1 in]
            n124 = Generate User Event(user event=w529, event data cluster=w528, error in=w527) -> (error out=w526:errorcluster)  [unwired: 1 out]
            n125 = Bundle By Name(cluster=w518, "ExperimentControlEvents"=w516) -> (w517:refnum<class "ExperimentRunner.lvclass">)
            n126 = Generate User Event(user event=w524, event data cluster=w533, error in=w526) -> (error out=w522:errorcluster)  [unwired: 1 out]
          }
          event #4 {
            # "select row of listbox"
            n127 = event-data() -> ("CtlRef"=w549:refnum<vi>, "Coords"=w555:T16)  [unwired: 1 in, 6 out]
            n128 = invoke class="LstBox (strict)" method="Point To Row"(reference=w549, error in=w543, "Point"=w555) -> (reference out=w553:refnum<vi>, error out=w552:errorcluster, "Row"=w545:i32)  [unwired: 4 in, 4 out]
            n129 = property class="LstBox (strict)"(reference=w553, error in=w552, "Value"=w545) -> (reference out=w550:refnum<vi>, error out=w551:errorcluster)
            n130 = Bundle By Name(cluster=w547, "scriptSelected"=w545) -> (w546:refnum<class "ExperimentRunner.lvclass">)
            n131 = Close Reference(reference=w550, error in (no error)=w551) -> (error out=w554:errorcluster)
          }
          event #5 {
            # "ADD A PATH"
            n132 = event-data() -> ()  [unwired: 1 in, 8 out]
            n133 = call "loadDPScript.vi"("error in (no error)"=w565, "ExperimentRunner in"=w568) -> ("error out"=w559:errorcluster, "ExperimentRunner out"=w563:refnum<class "ExperimentRunner.lvclass">)  [unwired: 8 in]
            n134 = call "refreshListBox.vi"("error in (no error)"=w559, "Listbox"=w561, "ExperimentRunner in"=w563) -> ("error out"=w558:errorcluster, "Listbox out"=w560:refnum<vi>, "ExperimentRunner out"=w562:refnum<class "ExperimentRunner.lvclass">)  [unwired: 6 in]
          }
          event #6 {
            n135 = event-data() -> ()  [unwired: 1 in, 8 out]
            n136 = call "removeDPScript.vi"("error in (no error)"=w579, "ExperimentRunner in"=w581) -> ("error out"=w572:errorcluster, "ExperimentRunner out"=w576:refnum<class "ExperimentRunner.lvclass">)  [unwired: 8 in]
            n137 = call "refreshListBox.vi"("error in (no error)"=w572, "Listbox"=w574, "ExperimentRunner in"=w576) -> ("error out"=w571:errorcluster, "Listbox out"=w573:refnum<vi>, "ExperimentRunner out"=w575:refnum<class "ExperimentRunner.lvclass">)  [unwired: 6 in]
          }
          event #7 {
            # "send nothing is blank path"
            # "open a script in script editor.\nby sending an open event with the path\nof the script."
            n138 = event-data() -> ()  [unwired: 1 in, 8 out]
            n139 = Unbundle By Name(w596) -> ("scriptSelected"=w589:i32, "PathArray"=w590:path[])
            n140 = Index Array(array=w590, index=w589) -> (element=w588:path)
            n141 = Equal?(x=w588, y=path "") -> (x = y?=w586:bool)
            n142 = case shown="False" w586 {
              tunnel: w593 -> [w607 _]
              tunnel: w594 -> [w606 w608]
              tunnel: [w598 w608] -> w592
              tunnel: w588 -> [w597 _]
              frame #0 {
                n143 = call-dynamic "getEvents.vi"("error in (no error)"=w606, "ScriptEdEvents in"=w607) -> ("error out"=w599:errorcluster, "eventsToScriptEd"=w605:T6, "ScriptEvent"=w603:refnum<user-event>)  [unwired: 6 in, 1 out]
                n144 = Unbundle By Name(w605) -> ("open"=w604:cluster{"Path":path})
                n145 = Bundle By Name(cluster=w604, "Path"=w597) -> (w601:cluster{"Path":path})
                n146 = Bundle("eventId"=enum16{"Open", "Save", "Close"}."Open", "open"=w601) -> (w600:T9)  [unwired: 1 in]
                n147 = Generate User Event(user event=w603, event data cluster=w600, error in=w599) -> (error out=w598:errorcluster)  [unwired: 1 out]
              }
              frame #1 {
              }
            }
          }
          event #8 {
            # "Run a Single Script"
            n148 = event-data() -> ()  [unwired: 1 in, 8 out]
            n149 = Unbundle By Name(w614) -> ("scriptSelected"=w617:i32)
            n150 = call "runSingleScriptV3.vi"("error in (no error)"=w615, "HWLoop"="HW Loop?", "index"=w617, "ExperimentRunner in"=w614) -> ("error out"=w611:errorcluster, "ExperimentRunner out"=w613:refnum<class "ExperimentRunner.lvclass">)  [unwired: 6 in]
          }
          event #9 {
            n151 = event-data() -> ()  [unwired: 1 in, 8 out]
            n152 = call "sendStop.vi"("error in (no error)"=w627, "stop"=enum16{"stopBeforeNext", "stopNow"}."stopNow" ("stop 2"), "ExperimentRunner in"=w625) -> ("error out"=w626:errorcluster, "ExperimentRunner out"=w624:refnum<class "ExperimentRunner.lvclass">)  [unwired: 7 in]
          }
          event #10 {
            n153 = event-data() -> ()  [unwired: 1 in, 8 out]
            n154 = Unbundle By Name(w646) -> ("deviceDataBaseConnection"=w642:refnum<class "deviceDataBase.lvclass">)
            n155 = call "isRunning.vi"("error in (no error)"=w635, "StaticOutputEditor in"=w637) -> ("error out"=w634:errorcluster, "running?"=w633:bool, "StaticOutputEditor out"=w636:refnum<class "StaticOutputEditor.lvclass">)  [unwired: 7 in]
            n156 = case shown="False" w633 {
              tunnel: w645 -> [w658 _]
              tunnel: [w657 w660] -> w644
              tunnel: [w656 w661] -> w643
              tunnel: w642 -> [w655 _]
              tunnel: w636 -> [w651 w662]
              tunnel: w635 -> [w649 w659]
              tunnel: w634 -> [w650 _]
              frame #0 {
                n157 = call "close.vi"("error in (no error)"=w650, "StaticOutputEditor in"=w651) -> ("error out"=w647:errorcluster, "StaticOutputEditor out"=w648:refnum<class "StaticOutputEditor.lvclass">)  [unwired: 8 in]
                n158 = call "getUnrestrictedChannelArray.vi"("error in (no error)"=w649, "deviceDataBase in"=w655) -> ("error out"=w653:errorcluster, "ChannelArray.lvclass"=w654:refnum<class "ChannelArray.lvclass">)  [unwired: 7 in, 1 out]
                n159 = call <vilib>:"Merge Errors.vi"("error in 2 (no error)"=w653, "error in 1 (no error)"=w647) -> ("error out"=w652:errorcluster)  [unwired: 5 in]
                n160 = call-dynamic "run.vi"("error in (no error)"=w652, "HWControllerEvents"=w658, "ChannelArray"=w654, "StaticOutputEditor"=w648) -> ("error out"=w657:errorcluster, "StaticOutputEditor out"=w656:refnum<class "StaticOutputEditor.lvclass">)  [unwired: 6 in]
              }
              frame #1 {
                n161 = call "showFrontEnd.vi"("error in (no error)"=w659, "StaticOutputEditor in"=w662) -> ("error out"=w660:errorcluster, "StaticOutputEditor out"=w661:refnum<class "StaticOutputEditor.lvclass">)  [unwired: 8 in]
              }
            }
          }
          event #11 {
            # "close compiler"
            # "Compiler"
            n162 = event-data() -> ()  [unwired: 1 in, 2 out]
            n163 = Unbundle By Name(w685) -> ("deviceDataBaseConnection"=w686:refnum<class "deviceDataBase.lvclass">, "HWControllerEvents"=w671:refnum<class "HWControllerEvents.lvclass">)
            n164 = Bundle(TRUE) -> (w677:cluster{bool})  [unwired: 1 in]
            n165 = Bundle("eventId"=T4."restartCompiler", w677) -> (w676:T17)  [unwired: 1 in]
            n166 = Generate User Event(user event=w679, event data cluster=w676, error in=w673) -> (error out=w672:errorcluster)  [unwired: 1 out]
            n167 = call "loadDatabase.vi"("error in (no error)"=w672, "deviceDataBase in"=w686) -> ("error out"=w669:errorcluster, "deviceDataBase out"=w670:refnum<class "deviceDataBase.lvclass">)  [unwired: 7 in, 1 out]
            n168 = call "close.vi"("error in (no error)"=w669, "Compiler in"=w668) -> ("error out"=w666:errorcluster, "Compiler out"=w667:refnum<class "Compiler.lvclass">)  [unwired: 8 in]
            n169 = call "databaseGF.vi"("deviceDataBase in"=w670, "Enum"=enum16{"write", "read"}."write") -> ()  [unwired: 9 in, 1 out]
            n170 = call "run.vi"("error in (no error)"=w666, "deviceDataBase"=w670, "HWControllerEvents"=w671, "Compiler in"=w667) -> ("error out"=w664:errorcluster, "Compiler out"=w665:refnum<class "Compiler.lvclass">)  [unwired: 6 in]
            n171 = Bundle By Name(cluster=w685, "deviceDataBaseConnection"=w670) -> (w684:refnum<class "ExperimentRunner.lvclass">)
          }
        }
      }
      n172 = call "isRunning.vi"("error in (no error)"=w24, "StaticOutputEditor in"=w25) -> ("error out"=w23:errorcluster, "running?"=w22:bool, "StaticOutputEditor out"=w21:refnum<class "StaticOutputEditor.lvclass">)  [unwired: 7 in]
      n173 = Close Reference(reference=w53, error in (no error)=w24) -> (error out=w43:errorcluster)
      n174 = case shown="False" w22 {
        tunnel: w23 -> [w54 w59]
        tunnel: w21 -> [w55 w58]
        tunnel: [w55 w57] -> w20
        tunnel: [w54 w56] -> w19
        frame #0 {
        }
        frame #1 {
          n175 = call "showFrontEnd.vi"("error in (no error)"=w59, "StaticOutputEditor in"=w58) -> ("error out"=w56:errorcluster, "StaticOutputEditor out"=w57:refnum<class "StaticOutputEditor.lvclass">)  [unwired: 8 in]
        }
      }
      n176 = Close Reference(reference=w44, error in (no error)=w43) -> (error out=w18:errorcluster)
      n177 = call "close.vi"("error in (no error)"=w19, "StaticOutputEditor in"=w20) -> ("error out"=w17:errorcluster)  [unwired: 8 in, 1 out]
      n178 = call <vilib>:"Merge Errors.vi"("error in 3 (no error)"=w17, "error in 1 (no error)"=w18) -> ("error out"=w41:errorcluster)  [unwired: 5 in]
    }
    frame #1 {
    }
  }
  "error out" <- w9
  "Views.lvlib:ExperimentControl.lvlib:ExperimentRunner out" <- w8
